vi "CLSUIP_OverrideErrMsgs.vi"() -> ()   [LabVIEW 2021, in "MemberVICreation.lvlib" / "VIRetooler.lvclass"]
uses:
  <resource>/Framework/Providers/LVClassLibrary/NewAccessors/VIRetooler/VIRetooler.lvclass
panel:
  in  "Conflicting Name Error":string="Unable to create a VI for override because of a name conflict. Two VIs with the same name cannot be in memory. Save or close the first VI with this name before creating the second."
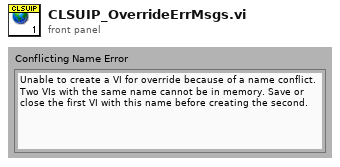
[diagram p1: front panel]
diagram:
